vi "Measure Rectangle Width.vi"(10 "Rect Bounding Box":T1, 11 "Refnum in":T2(plugin-control)) -> (1 "Width":i32, 3 "Refnum out":T2(plugin-control))   [LabVIEW 2013]
uses:
  <vilib>/vision/NI_Vision_Development_Module.lvlib
panel:
  out "Bounding Box Width":i32
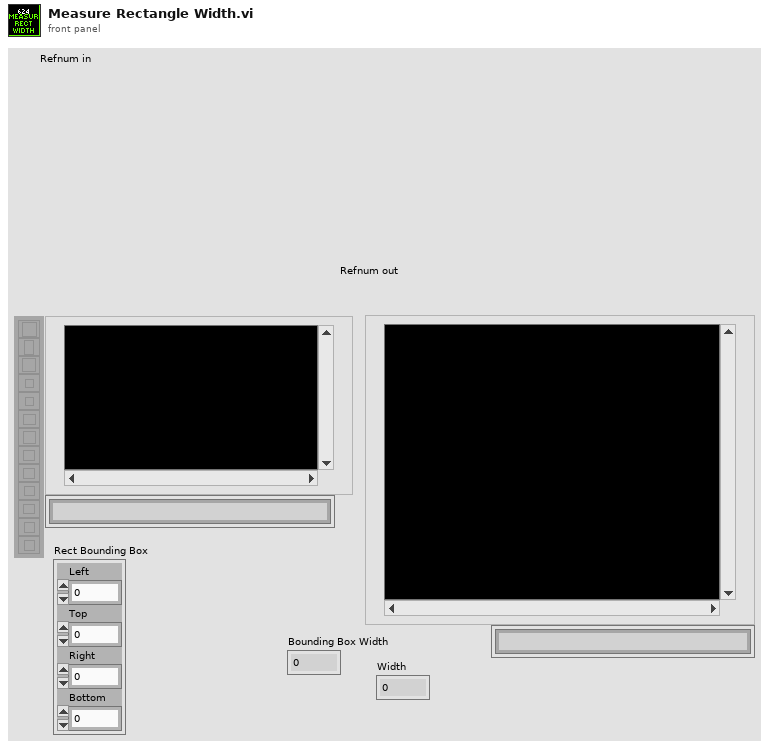
[diagram p1: front panel]
types:
  T1 = cluster{"Left":dbl, "Top":dbl, "Right":dbl, "Bottom":dbl}
  T2 = typedef "IMAQ Image.ctl" = refnum<image>
  T3 = typedef "Image Type" = u32
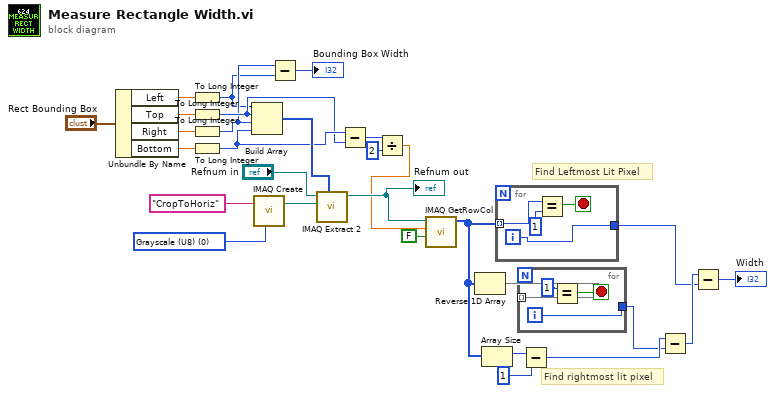
[diagram p0: block diagram]
diagram:
  w28 = T3 0 items=["Grayscale (U8)", "Grayscale (I16)", "Grayscale (SGL)", "Complex (CSG)", "RGB (U32)", "HSL (U32)", "RGB (U64)", "Grayscale (U16)"] ("Image Type")
  # "Find rightmost lit pixel"
  # "Find Leftmost Lit Pixel"
  n1 = Unbundle By Name("Rect Bounding Box") -> ("Left"=w21:dbl, "Top"=w22:dbl, "Right"=w23:dbl, "Bottom"=w24:dbl)
  n2 = To Long Integer(number=w21) -> (32bit integer=w2:i32)
  n3 = To Long Integer(number=w22) -> (32bit integer=w17:i32)
  n4 = To Long Integer(number=w23) -> (32bit integer=w3:i32)
  n5 = To Long Integer(number=w24) -> (32bit integer=w18:i32)
  n6 = Build Array(w2, w17, w3, w18) -> (w25:i32[])
  n7 = call "IMAQ Create"("Image Name"="CropToHoriz", "Image Type"=w28) -> ("New Image"=w27:T2)  [unwired: 3 in, 1 out]
  n8 = Subtract(x=w3, y=w2) -> (x-y=→"Bounding Box Width":i32)
  n9 = call "IMAQ Extract 2"("Optional Rectangle"=w25, "Image Dst"=w27, "Image Src"="Refnum in") -> ("Image Dst Out"=w19:T2)  [unwired: 7 in, 1 out]
  "Refnum out" <- w19
  n10 = Subtract(x=w18, y=w17) -> (x-y=w16:i32)
  n11 = Divide(x=w16, y=2) -> (x/y=w14:dbl)
  n12 = call "IMAQ GetRowCol"("Image"=w19, "Number"=w14, "Row / Column (Row)"=FALSE) -> ("Pixels (U8)"=w11:u8[])  [unwired: 3 in, 4 out]
  n13 = Reverse 1D Array(array=w11) -> (reversed array=w12:u8[])
  n14 = Array Size(array=w11) -> (size(s)=w10:i32)
  n15 = for {
    tunnel: w11 -> [w33] mode=indexing
    tunnel: [w31] -> w5
    i -> [w31]
    stop <- w30 stop-if-true
    n16 = Equal?(x=w33, y=u8 1) -> (x = y?=w30:bool)
  }
  n17 = for {
    tunnel: w12 -> [w37] mode=indexing
    tunnel: [w34] -> w7
    i -> [w34]
    stop <- w35 stop-if-true
    n18 = Equal?(x=u8 1, y=w37) -> (x = y?=w35:bool)
  }
  n19 = Subtract(x=w10, y=1) -> (x-y=w8:i32)
  n20 = Subtract(x=w8, y=w7) -> (x-y=w6:i32)
  n21 = Subtract(x=w6, y=w5) -> (x-y=→"Width":i32)
